vi "StandDev.vi"() -> ()   [LabVIEW 2022 SP3]
panel:
  out "sigi":dbl format="%.2f"
  out "sigm":dbl format="%.2f"
  out "sigb":dbl format="%.2f"
  out "sigI":dbl format="%.2f"
  out "sigm":dbl format="%.2f"
  out "sigb":dbl format="%.2f"
  in  "TPI cells":dbl=1.0 format="%.2f"
  in  "#lines":dbl=33.0 format="%.2f"
  in  "bandwidth":dbl=4.5 format="%.2f"
  out "N (spec cells)":dbl format="%.2f"
  in  "center freq":dbl=5.75 format="%.2f"
  in  "#RF pts":dbl=64.0 format="%.2f"
  # "TPI"
  # "ROI"
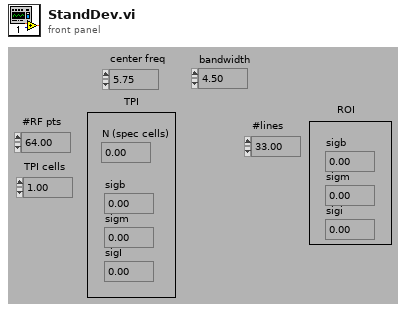
[diagram p1: front panel]
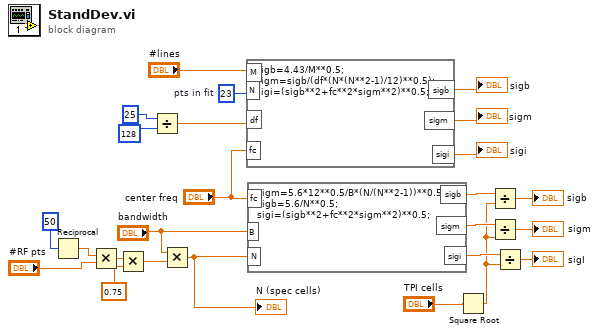
[diagram p0: block diagram]
diagram:
  w8 = 23  # pts in fit
  n1 = Reciprocal(x=50) -> (1/x=w11:dbl)
  n2 = Multiply(x=w11, y="#RF pts") -> (x*y=w25:dbl)
  n3 = Multiply(x=w25, y=0.75) -> (x*y=w23:dbl)
  n4 = Divide(x=25, y=128) -> (x/y=w12:dbl)
  n5 = Multiply(x="bandwidth", y=w23) -> (x*y=w22:dbl)
  "N (spec cells)" <- w22
  n6 = formula code="sigb=4.43/M**0.5;\nsigm=sigb/(df*(N*(N**2-1)/12)**0.5);\nsigi=(sigb**2+fc**2*sigm**2)**0.5;"("N"=w8, "fc"="center freq", "df"=w12, "M"="#lines") -> ("sigb"=→"sigb":dbl, "sigm"=→"sigm":dbl, "sigi"=→"sigi":dbl)
  n7 = formula code="sigm=5.6*12**0.5/B*(N/(N**2-1))**0.5;\nsigb=5.6/N**0.5;\nsigi=(sigb**2+fc**2*sigm**2)**0.5;"("B"="bandwidth", "N"=w22, "fc"="center freq") -> ("sigb"=w18:dbl, "sigm"=w17:dbl, "sigi"=w3:dbl)
  n8 = Square Root(x="TPI cells") -> (sqrt(x)=w1:dbl)
  n9 = Divide(x=w18, y=w1) -> (x/y=→"sigb":dbl)
  n10 = Divide(x=w17, y=w1) -> (x/y=→"sigm":dbl)
  n11 = Divide(x=w3, y=w1) -> (x/y=→"sigI":dbl)
